vi "Write Self ID.vi"(10 "self-id":string, 11 "Properties in":refnum<class "Properties.lvclass">) -> (3 "Properties out":refnum<class "Properties.lvclass">)   [LabVIEW 2020, in "Caraya.lvlib" / "Properties.lvclass"]
uses:
  Properties.lvclass
  Properties.lvclass/Properties.ctl
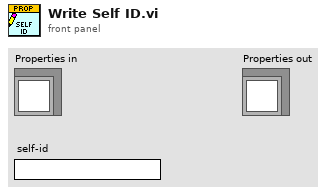
[diagram p1: front panel]
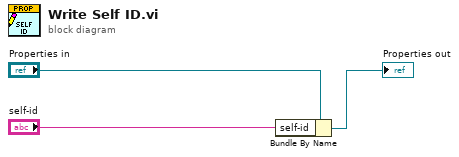
[diagram p0: block diagram]
diagram:
  n1 = Bundle By Name(cluster="Properties in", "self-id"="self-id") -> (→"Properties out":refnum<class "Properties.lvclass">)
